vi "VMI_create_image_from_points.vi"(2 "New Array":bool, 3 "Image Info":T1={"X size"=782.0, "Y size"=582.0, "Centroiding"=1.0}, 4 "Input array":i16[][](array[numeric]), 5 "Points":cluster{"X":sgl, "Y":sgl}[](array[cluster])=array[24000 elements]) -> (1 "Image Array":i16[][](array[numeric]))   [LabVIEW 2018]
uses:
  Type defs/Image_info.ctl
panel:
  out "Intensity Graph 2":i16[][](graph)
  out "sum":i32
  out "Numeric":i32
  out "size(s)":i32
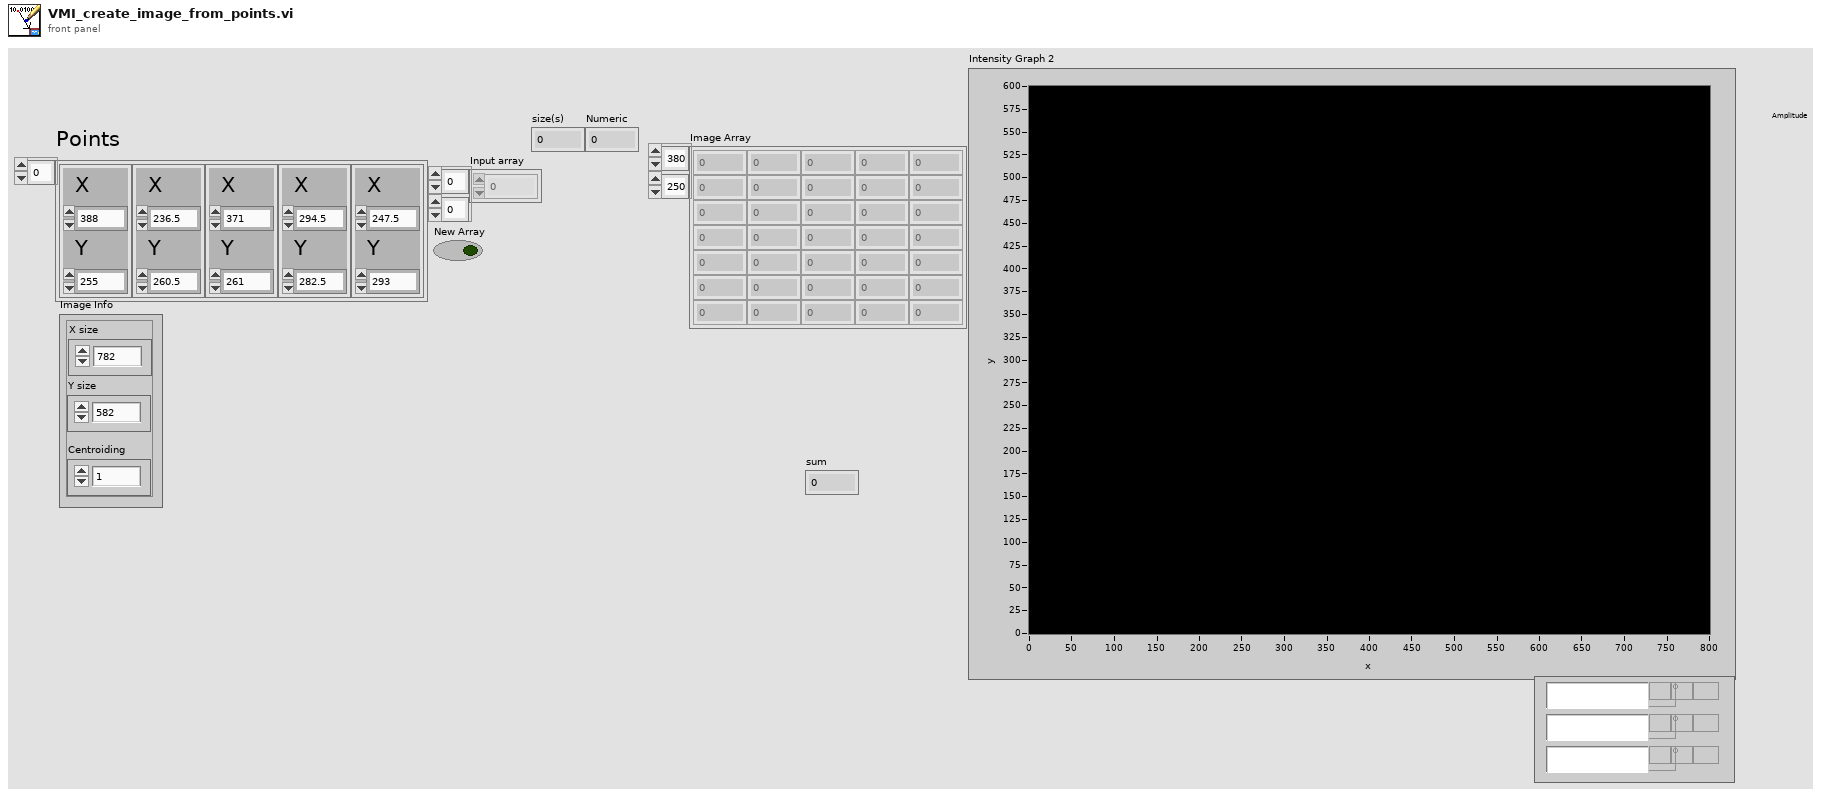
[diagram p1: front panel]
types:
  T1 = typedef "Image_info.ctl" = cluster{"X size":dbl, "Y size":dbl, "Centroiding":dbl}
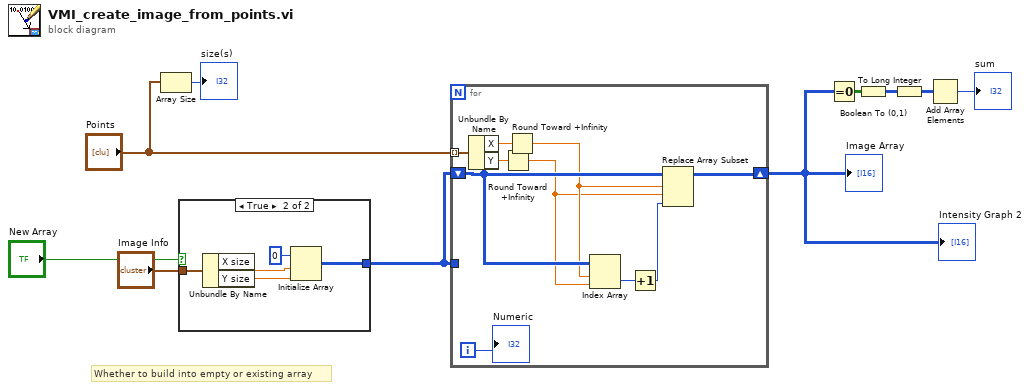
[diagram p0: block diagram]
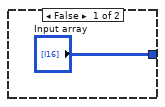
[diagram p2: hidden frame]
diagram:
  # "Whether to build into empty or existing array"
  n1 = Array Size(array="Points") -> (size(s)=→"size(s)":i32)
  n2 = case shown="True" "New Array" {
    tunnel: "Image Info" -> [_ w15]
    tunnel: ["Input array" w12] -> w4
    frame False {
    }
    frame True {
      n3 = Unbundle By Name(w15) -> ("X size"=w14:dbl, "Y size"=w13:dbl)
      n4 = Initialize Array(i16 0 ("element"), w14, w13) -> (w12:i16[][])
    }
  }
  n5 = for {
    tunnel: "Points" -> [w26] mode=indexing
    tunnel: w4 -> [_]
    shift-right: [w21] -> w1
    shift-left: w4 -> [w19]
    i -> [w20]
    n6 = Unbundle By Name(w26) -> ("X"=w25:sgl, "Y"=w24:sgl)
    n7 = Round Toward +Infinity(x=w24) -> (ceil(x): smallest int >= x=w17:sgl)
    n8 = Round Toward +Infinity(x=w25) -> (ceil(x): smallest int >= x=w18:sgl)
    n9 = Index Array(array=w19, index (row)=w18, index (col)=w17) -> (element=w23:i16)
    n10 = Increment(x=w23) -> (x+1=w22:i16)
    n11 = Replace Array Subset(array=w19, new element=w22, index (row)=w18, index (col)=w17) -> (w21:i16[][])
    "Numeric" <- w20
  }
  "Image Array" <- w1
  "Intensity Graph 2" <- w1
  n12 = Equal To 0?(x=w1) -> (x = 0?=w8:bool[][])
  n13 = Boolean To (0,1)(Boolean=w8) -> (0, 1=w7:i16[][])
  n14 = To Long Integer(number=w7) -> (32bit integer=w6:i32[][])
  n15 = Add Array Elements(numeric array=w6) -> (sum=→"sum":i32)
